vi "niDTS WLAN INSTR RX Configure Payload.vi"(8 "error in (no error)":errorcluster, 11 "niDTS WLAN INSTR RX in":refnum<class "niDTS WLAN INSTR RX.lvclass">) -> (0 "error out":errorcluster, 3 "niDTS WLAN INSTR RX out":refnum<class "niDTS WLAN INSTR RX.lvclass">)   [LabVIEW 2015, in "niDTS WLAN.lvlib" / "niDTS WLAN INSTR RX.lvclass"]
doc: "Sets:\n\n* PayloadLength"
uses:
  niDTS WLAN INSTR RX.lvclass
  niDTS WLAN INSTR RX.lvclass/niDTS WLAN INSTR RX.ctl
  RiviInstDriver/niRfsgWlan/Objects/niRfsgWlan.lvclass
  niDTS WLAN.lvlib
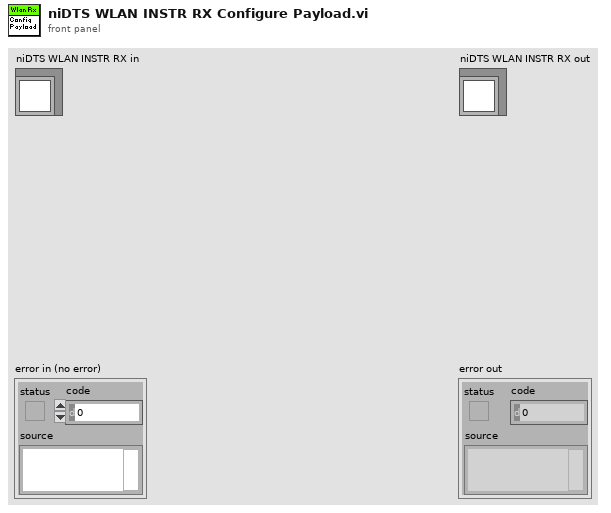
[diagram p1: front panel]
types:
  T1 = typedef "niDTS WLAN.lvlib/niDTS WLAN INC Standard.ctl" = enum16{"802.11 b DSSS", "802.11 a/g OFDM", "802.11 n HT", "802.11 ac VHT"}
  T2 = typedef "niDTS WLAN.lvlib/niDTS WLAN INC DSSS Data Rate.ctl" = enum16{"1", "2", "5.5", "11"}
  T3 = typedef "niDTS WLAN.lvlib/niDTS WLAN INC OFDM Data Rate.ctl" = enum16{"6", "9", "12", "18", "24", "36", "48", "54"}
  T4 = typedef "niDTS WLAN.lvlib/niDTS WLAN INC Type.ctl" = enum16{"b - 1 Mbps", "b - 2 Mbps", "b - 5.5 Mbps", "b - 11 Mbps", "ag - 6 Mbps", "ag - 9 Mbps", "ag - 12 Mbps", "ag - 18 Mbps", "ag - 24 Mbps", "ag - 36 Mbps", "ag - 48 Mbps", "ag - 54 Mbps", "n - MCS0", "n - MCS1", "n - MCS2", "n - MCS3", "n - MCS4", "n - MCS5", "n - MCS6", "n - MCS7", "n - MCS8", "n - MCS9", "n - MCS10", "n - MCS11", "n - MCS12", "n - MCS13", "n - MCS14", "n - MCS15", "n - MCS16", "n - MCS17", "n - MCS18", "n - MCS19", "n - MCS20", "n - MCS21", "n - MCS22", "n - MCS23", "n - MCS24", "n - MCS25", "n - MCS26", "n - MCS27", "n - MCS28", "n - MCS29", "n - MCS30", "n - MCS31", "ac - MCS0 -1", "ac - MCS1 -1", "ac - MCS2 -1", "ac - MCS3 -1", "ac - MCS4 -1", "ac - MCS5 -1", "ac - MCS6 -1", "ac - MCS7 -1", "ac - MCS8 -1", "ac - MCS9 -1", "ac - MCS0 -2", "ac - MCS1 -2", "ac - MCS2 -2", "ac - MCS3 -2", "ac - MCS4 -2", "ac - MCS5 -2", "ac - MCS6 -2", "ac - MCS7 -2", "ac - MCS8 -2", "ac - MCS9 -2", "ac - MCS0 -3", "ac - MCS1 -3", "ac - MCS2 -3", "ac - MCS3 -3", "ac - MCS4 -3", "ac - MCS5 -3", "ac - MCS6 -3", "ac - MCS7 -3", "ac - MCS8 -3", "ac - MCS9 -3", "ac - MCS0 -4", "ac - MCS1 -4", "ac - MCS2 -4", "ac - MCS3 -4", "ac - MCS4 -4", "ac - MCS5 -4", "ac - MCS6 -4", "ac - MCS7 -4", "ac - MCS8 -4", "ac - MCS9 -4"}
  T5 = typedef "niRfsgWlan.lvclass/niRfsgWlan INC Handle.ctl" = refnum<data-value>
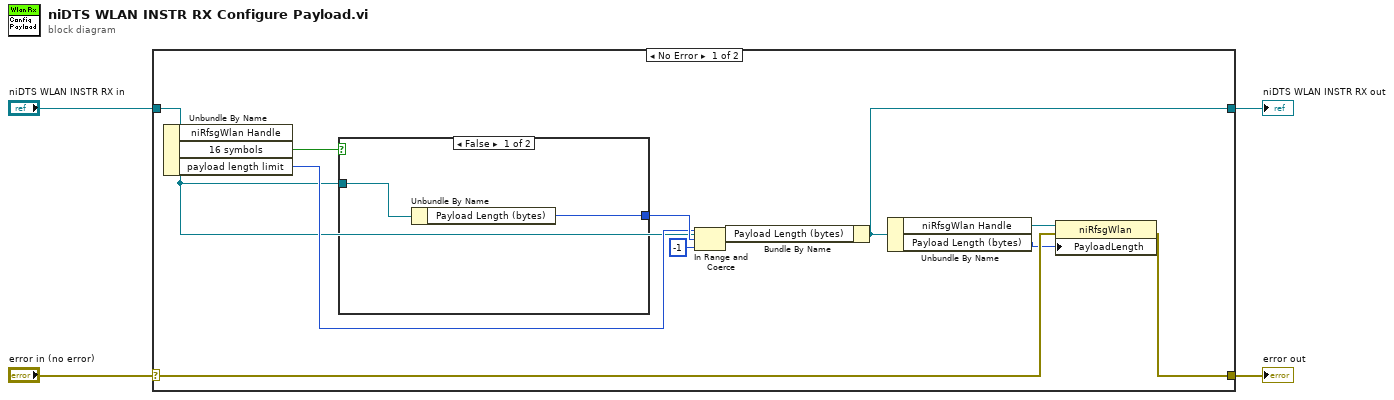
[diagram p0: block diagram]
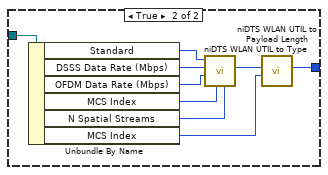
[diagram p2: hidden frame]
diagram:
  n1 = case shown="No Error" "error in (no error)" {
    selector: "error in (no error)" -> [w8 w28]
    tunnel: [w7 w28] -> w3
    tunnel: [w10 w27] -> w1
    tunnel: "niDTS WLAN INSTR RX in" -> [w11 w27]
    frame No Error {
      n2 = Unbundle By Name(w11) -> ("16 symbols"=w5:bool, "payload length limit"=w12:i32)  [unwired: 1 out]
      n3 = case shown="False" w5 {
        tunnel: w11 -> [w16 w19]
        tunnel: [w17 w18] -> w14
        frame False {
          n4 = Unbundle By Name(w16) -> ("Payload Length (bytes)"=w17:i32)
        }
        frame True {
          n5 = Unbundle By Name(w19) -> ("Standard"=w26:T1, "DSSS Data Rate (Mbps)"=w25:T2, "OFDM Data Rate (Mbps)"=w24:T3, "MCS Index"=w23:i32, "N Spatial Streams"=w22:i32, "MCS Index"=w20:i32)
          n6 = call "niDTS WLAN UTIL to Type.vi"("N_SS"=w22, "MCS"=w23, "OFDM Data Rate (Mbps)"=w24, "DSSS Data Rate (Mbps)"=w25, "Standard"=w26) -> ("WLAN Type"=w21:T4)  [unwired: 6 in]
          n7 = call "niDTS WLAN UTIL to Payload Length.vi"("CH BW"=w20, "WLAN Type"=w21) -> ("Payload Length"=w18:i32)  [unwired: 9 in]
        }
      }
      n8 = In Range and Coerce(upper limit=w12, x=w14, lower limit=-1) -> (coerced(x)=w15:i32)  [unwired: 1 out]
      n9 = Bundle By Name(cluster=w11, "Payload Length (bytes)"=w15) -> (w10:refnum<class "niDTS WLAN INSTR RX.lvclass">)
      n10 = Unbundle By Name(w10) -> ("niRfsgWlan Handle"=w9:T5, "Payload Length (bytes)"=w6:i32)
      n11 = property class="niRfsgWlan"(reference=w9, error in=w8, "PayloadLength"=w6) -> (error out=w7:errorcluster)  [unwired: 1 out]
    }
    frame Error {
    }
  }
  "error out" <- w3
  "niDTS WLAN INSTR RX out" <- w1
